vi "XY Graph Normalize Plot.vi"(8 "Error In":errorcluster, 9 "Normalization Factor (Max *)":dbl=nan, 10 "Subtract Baseline? (No)":bool, 11 "Plot in":cluster{"X Array":dbl[], "Y Array":dbl[]}) -> (0 "Error Out":errorcluster, 3 "Plot out":cluster{"X Array":dbl[], "Y Array":dbl[]})   [LabVIEW 2021, in "XY Graph Add-Ons.lvlib"]
doc: "If <B>Subtract Baseline</B> is True, first subtract the minimum to the array.\n\nIf <B>Normalization Factor</B> is not connected (or NaN), divides the decay <B>Y Array</B> by its maximum (or max - min if <B>Subtract Baseline</B> is True).\n\nIf <B>Normalization Factor</B> is connected, divide the decay <B>Y Array</B> by this factor. Typically, this would be the number of pixels in a ROI, in order to obtain a \"per-pixel\" decay."
uses:
  XY Graph Add-Ons.lvlib
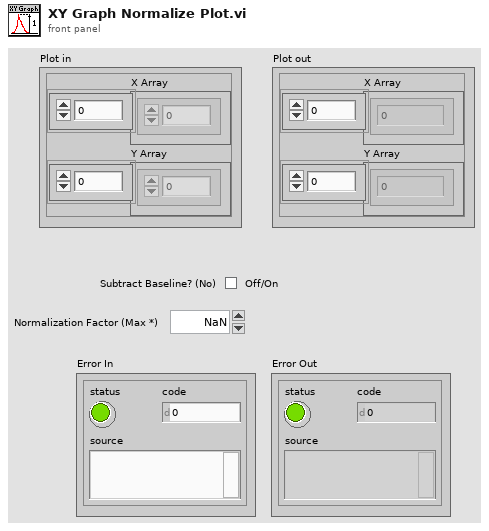
[diagram p1: front panel]
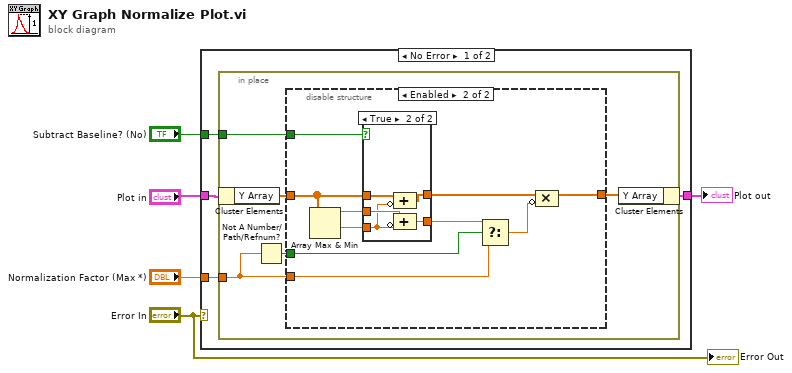
[diagram p0: block diagram]
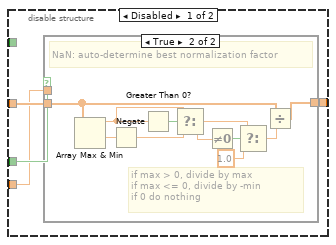
[diagram p2: hidden frame]
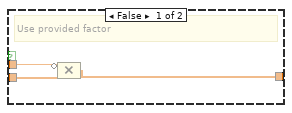
[diagram p3: hidden frame]
diagram:
  n1 = case shown="No Error" "Error In" {
    tunnel: "Plot in" -> [w9 w49]
    tunnel: [w8 w49] -> w4
    tunnel: "Normalization Factor (Max *)" -> [w7 _]
    tunnel: "Subtract Baseline? (No)" -> [w6 _]
    frame No Error {
      n2 = in-place {
        in-place-border: w7 -> [w11]
        in-place-border: w6 -> [w10]
        n3 = in-place-cluster #1(w9) -> ("Y Array"=w14:dbl[])
        n4 = Not A Number/Path/Refnum?(number/path/refnum=w11) -> (NaN/Path/Refnum?=w12:bool)
        n5 = disable-structure shown="Enabled" {
          disable-tunnel: w14 -> [w18 w40]
          disable-tunnel: [w17 w36] -> w13
          disable-tunnel: w12 -> [w16 w34]
          disable-tunnel: w11 -> [w15 w33]
          disable-tunnel: w10 -> [_ w41]
          frame Disabled {
            n6 = case shown="True" w16 {
              tunnel: w18 -> [w21 w27]
              tunnel: [w19 w26] -> w17
              tunnel: w15 -> [w20 _]
              frame False {
                # "Use provided factor"
                n7 = Compound Arithmetic op=MULTIPLY(invert w20, w21) -> (w19:dbl[])
              }
              frame True {
                # "if max > 0, divide by max\nif max <= 0, divide by -min\nif 0 do nothing"
                # "NaN: auto-determine best normalization factor"
                n8 = Array Max & Min(array=w27) -> (max value=w30:dbl, min value=w28:dbl)  [unwired: 2 out]
                n9 = Negate(x=w28) -> (-x=w29:dbl)
                n10 = Greater Than 0?(x=w30) -> (x > 0?=w31:bool)
                n11 = Select(t=w30, s=w31, f=w29) -> (s? t:f=w23:dbl)
                n12 = Not Equal To 0?(x=w23) -> (x != 0?=w25:bool)
                n13 = Select(t=w23, s=w25, f=1.0) -> (s? t:f=w24:dbl)
                n14 = Divide(x=w27, y=w24) -> (x/y=w26:dbl[])
              }
            }
          }
          frame Enabled {
            n15 = Array Max & Min(array=w40) -> (max value=w38:dbl, min value=w39:dbl)  [unwired: 2 out]
            n16 = case shown="True" w41 {
              tunnel: w40 -> [w43 w48]
              tunnel: w39 -> [_ w46]
              tunnel: w38 -> [w42 w47]
              tunnel: [w43 w45] -> w37
              tunnel: [w42 w44] -> w35
              frame False {
              }
              frame True {
                n17 = Compound Arithmetic op=ADD(w48, invert w46) -> (w45:dbl[])
                n18 = Compound Arithmetic op=ADD(w47, invert w46) -> (w44:dbl)
              }
            }
            n19 = Select(t=w35, s=w34, f=w33) -> (s? t:f=w32:dbl)
            n20 = Compound Arithmetic op=MULTIPLY(w37, invert w32) -> (w36:dbl[])
          }
        }
        n21 = in-place-cluster #1("Y Array"=w13) -> (w8:cluster{"X Array":dbl[], "Y Array":dbl[]})
      }
    }
    frame Error {
    }
  }
  "Plot out" <- w4
  "Error Out" <- "Error In"
